vi "2016-120_Shutdown and close PS.vi"(6 "Current Limit (0)":dbl=3.0 min=0.0 max=6.0 format="%#.2g", 8 "error in":errorcluster, 9 "Output Voltage (0)":dbl min=0.0 max=18.0 format="%#.2f", 10 "Maximum Output Voltage (18)":dbl=32.0 min=0.0 max=72.0 format="%#.2f", 11 "Com Port":string) -> (0 "error out":errorcluster, 3 "VISA resource name out":refnum<visa-resource-name>="COM7")   [LabVIEW 2015]
uses:
  <instrlib>/BK Precision 178XB Series/BK Precision 178XB Series.lvlib
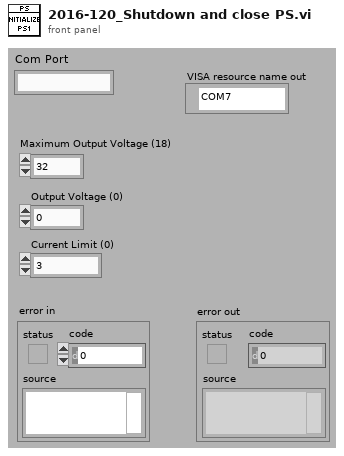
[diagram p1: front panel]
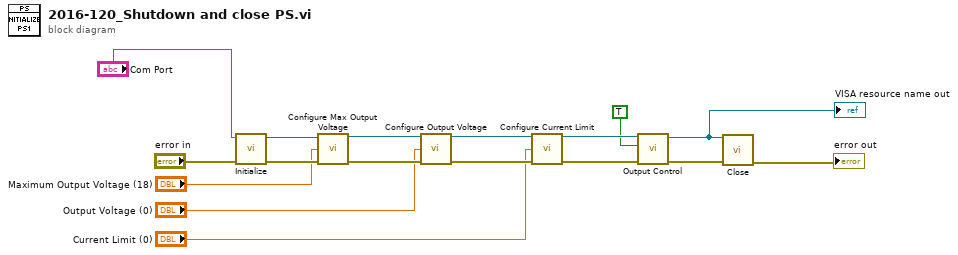
[diagram p0: block diagram]
diagram:
  n1 = call <instrlib>:"Initialize.vi"("error in (no error)"="error in", "VISA resource name"="Com Port") -> ("error out"=w16:errorcluster, "VISA resource name out"=w17:refnum<visa-resource-name>)  [unwired: 8 in]
  n2 = call <instrlib>:"Configure Max Output Voltage.vi"("VISA resource name"=w17, "Maximum Output Voltage (18)"="Maximum Output Voltage (18)", "error in (no error)"=w16) -> ("VISA resource name out"=w15:refnum<visa-resource-name>, "error out"=w12:errorcluster)  [unwired: 11 in]
  n3 = call <instrlib>:"Configure Output Voltage.vi"("VISA resource name"=w15, "Output Voltage (0)"="Output Voltage (0)", "error in (no error)"=w12) -> ("VISA resource name out"=w14:refnum<visa-resource-name>, "error out"=w13:errorcluster)  [unwired: 11 in]
  n4 = call <instrlib>:"Configure Current Limit.vi"("VISA resource name"=w14, "Current Limit (0)"="Current Limit (0)", "error in (no error)"=w13) -> ("VISA resource name out"=w11:refnum<visa-resource-name>, "error out"=w10:errorcluster)  [unwired: 11 in]
  n5 = call <instrlib>:"Output Control.vi"("error in (no error)"=w10, "Enable Output Terminals (F: Off)"=TRUE, "VISA resource name"=w11) -> ("error out"=w3:errorcluster, "VISA resource name out"=w2:refnum<visa-resource-name>)  [unwired: 7 in]
  "VISA resource name out" <- w2
  n6 = call <instrlib>:"Close.vi"("error in (no error)"=w3, "VISA resource name"=w2) -> ("error out"=→"error out":errorcluster)  [unwired: 9 in]
